vi "RunDigitalStimTicklish.vi"(3 "error in (no error)":errorcluster, 4 "digital stimuli":T2(array[cluster]), 5 "Serial USB port name":refnum<visa-resource-name>) -> (0 "error out":errorcluster, 1 "time-sync":T1, 2 "Serial USB port name out":refnum<visa-resource-name>)   [LabVIEW 2015]
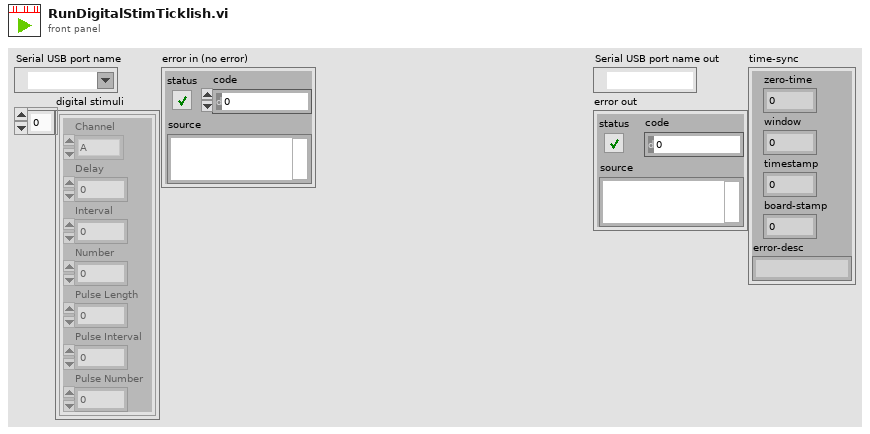
[diagram p1: front panel]
types:
  T1 = cluster{"zero-time":dbl, "window":dbl, "timestamp":dbl, "board-stamp":dbl, "error-desc":string}
  T2 = cluster{"Channel":enum16{"A", "B", "C", "D", "E", "F", "G", "H", "I", "J", "K", "L", "M", "N", "O", "P", "Q", "R", "S", "T", "U", "V", "W", "X"}, "Delay":dbl, "Interval":dbl, "Number":i32, "Pulse Length":dbl, "Pulse Interval":dbl, "Pulse Number":i32}[]
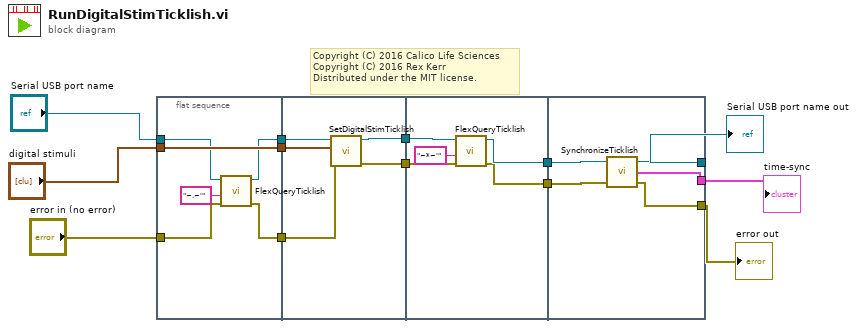
[diagram p0: block diagram]
diagram:
  # "Copyright (C) 2016 Calico Life Sciences\nCopyright (C) 2016 Rex Kerr\nDistributed under the MIT license."
  n1 = flat-sequence {
    tunnel: "error in (no error)" -> [w16]
    tunnel: "digital stimuli" -> [w19]
    tunnel: "Serial USB port name" -> [w18]
    tunnel: [w17] -> w3
    tunnel: [w19] -> w2
    tunnel: [w15] -> w1
    tunnel: [w21] -> w10
    tunnel: [w20] -> w9
    tunnel: w3 -> [w24]
    tunnel: w2 -> [w23]
    tunnel: w1 -> [w22]
    tunnel: w10 -> [w29]
    tunnel: w9 -> [w28]
    tunnel: [w26] -> w8
    tunnel: [w25] -> w7
    tunnel: w8 -> [w34]
    tunnel: w7 -> [w33]
    tunnel: [w32] -> w6
    tunnel: [w31] -> w5
    tunnel: [w30] -> w4
    frame #0 {
      n2 = call "FlexQueryTicklish.vi"("error in (no error)"=w16, "write buffer"="~.~'", "Serial USB port name"=w18) -> ("error out"=w15:errorcluster, "Serial USB port name out"=w17:refnum<visa-resource-name>)  [unwired: 6 in, 1 out]
    }
    frame #1 {
      n3 = call "SetDigitalStimTicklish.vi"("error in (no error)"=w22, "digital stimuli"=w23, "Serial USB port name"=w24) -> ("error in (no error) 2"=w20:errorcluster, "Serial USB port name 2"=w21:refnum<visa-resource-name>)  [unwired: 7 in]
    }
    frame #2 {
      n4 = call "FlexQueryTicklish.vi"("error in (no error)"=w28, "write buffer"="~*~'", "Serial USB port name"=w29) -> ("error out"=w25:errorcluster, "Serial USB port name out"=w26:refnum<visa-resource-name>)  [unwired: 6 in, 1 out]
    }
    frame #3 {
      n5 = call "SynchronizeTicklish.vi"("error in (no error)"=w33, "Serial USB port name"=w34) -> ("error out"=w31:errorcluster, "time-sync"=w30:T1, "Serial USB port name out"=w32:refnum<visa-resource-name>)  [unwired: 1 in]
    }
  }
  "Serial USB port name out" <- w6
  "error out" <- w5
  "time-sync" <- w4
